vi "HW_GEN - Read Channel Default Parameters from XML File.vi"(8 "error in":errorcluster caption="错误输入（无错误）", 10 "ChanType":string="AI_QX", 11 "path to XML document":path=path "E:/00. 系统集成/!00000/11所 热气台等/SourceCodes/Builds/Files/CHdef.xml" caption="XML文档路径") -> (0 "错误输出":errorcluster, 2 "Chan dflt Para out":T3)   [LabVIEW 2016]
uses:
  Ctrls/HardWare _ Channel Configurations PopUp Type.ctl
  ToolKit/Popup/Private/Ctrls/POP_Data Type.ctl
  <vilib>/xml/Load XML File.vi
  <vilib>/xml/NI_XML.lvlib
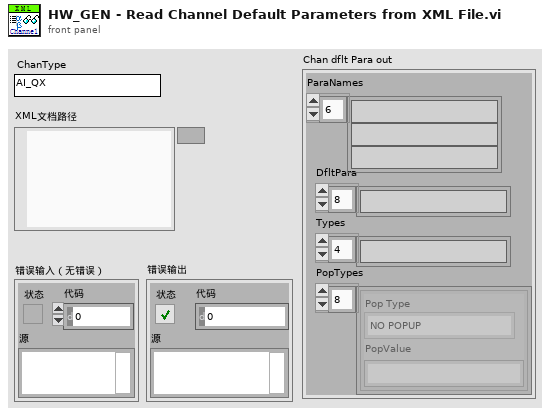
[diagram p1: front panel]
types:
  T1 = typedef "HardWare _ Channel Configurations PopUp Type.ctl" = cluster{"Pop Type":T2, "PopValue":string}
  T2 = typedef "POP_Data Type.ctl" = enum16{"NO POPUP", "Unkown", "String", "Integer", "Float", "Color", "Boolean", "Ring", "Captioned String", "Captioned Integer", "Button Color", "2 Int Cluster", "4 Int Cluster", "6-Dbl Cluster", "Path", "Combox", "Time", "ShotCut String"}
  T3 = cluster{"ParaNames":string[], "DfltPara":string[], "Types":string[], "PopTypes":T1[]}
  T4 = cluster{"Names":string[], "DfltValues":string[], "Types":string[], "PopTypes":T1[]}
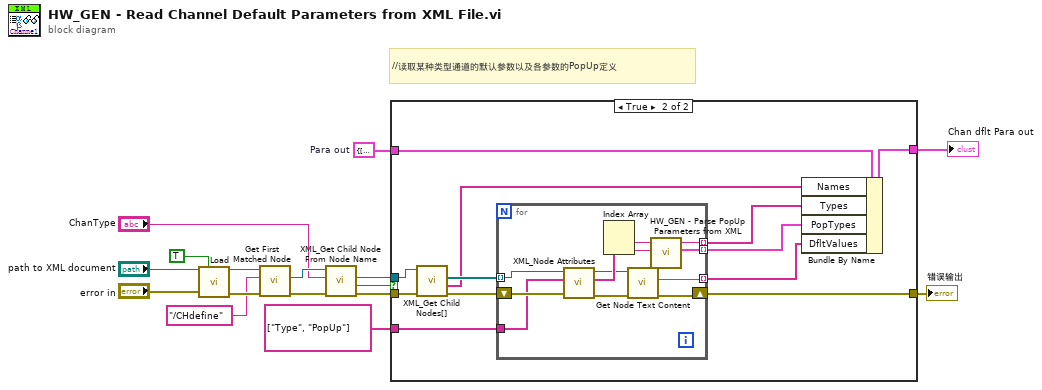
[diagram p0: block diagram]
diagram:
  w3 = T4 {"Names"=[], "DfltValues"=[], "Types"=[], "PopTypes"=[]}  # Para out
  # "//读取某种类型通道的默认参数以及各参数的PopUp定义"
  n1 = call-poly <vilib>:"Load.vi"("path to XML document"="path to XML document", "preserve whitespace (True)"=TRUE, "error in (no error)"="error in") -> ("DOM document out"=w12:refnum<k20>, "error out"=w14:errorcluster)  [unwired: 10 in, 1 out]
  n2 = call <vilib>:"Get First Matched Node.vi"("error in (no error)"=w14, "XPath expression"="/CHdefine", "node in"=w12) -> ("error out"=w10:errorcluster, "node result"=w11:refnum<k20>)  [unwired: 6 in, 1 out]
  n3 = call "XML_Get Child Node From Node Name.vi"("error in"=w10, "NodeName"="ChanType", "ref in"=w11) -> ("错误输出"=w5:errorcluster, "find?"=w7:bool, "subNode out"=w6:refnum<k20>)  [unwired: 6 in]
  n4 = case shown="True" w7 {
    tunnel: w6 -> [_ w29]
    tunnel: w5 -> [w17 w30]
    tunnel: string[] ["Type", "PopUp"] ("AttributeNames") -> [_ w26]
    tunnel: w3 -> [w18 w25]
    tunnel: [w18 w20] -> w2
    tunnel: [w17 w19] -> w1
    frame False {
    }
    frame True {
      n5 = call "XML_Get Child Nodes[].vi"("错误输入（无错误）"=w30, "ref in"=w29) -> ("错误输出"=w27:errorcluster, "NodeNames[]"=w24:string[], "ElementChildNod[]"=w28:refnum<k20>[])  [unwired: 6 in, 1 out]
      n6 = for {
        tunnel: w28 -> [w40] mode=indexing
        tunnel: w26 -> [w39]
        shift-right: [w35] -> w19
        shift-left: w27 -> [w41]
        tunnel: [w34] -> w21 mode=indexing
        tunnel: [w33] -> w23 mode=indexing
        tunnel: [w31] -> w22 mode=indexing
        n7 = call "XML_Node Attributes.vi"("error in"=w41, "AttributeNames"=w39, "node in"=w40) -> ("error out"=w36:errorcluster, "Values"=w38:string[], "node out"=w37:refnum<k20>)  [unwired: 6 in]
        n8 = Index Array(array=w38) -> (element #1=w33:string, element #2=w32:string)  [unwired: 2 in]
        n9 = call <vilib>:"Get Node Text Content.vi"("error in (no error)"=w36, "node in"=w37) -> ("error out"=w35:errorcluster, "node text"=w34:string)  [unwired: 7 in, 1 out]
        n10 = call "HW_GEN - Parse PopUp Parameters from XML.vi"("string in"=w32) -> ("PopUp"=w31:cluster{"Pop Type":T2, "string in":string})  [unwired: 10 in]
      }
      n11 = Bundle By Name(cluster=w25, "Names"=w24, "Types"=w23, "PopTypes"=w22, "DfltValues"=w21) -> (w20:T4)
    }
  }
  "Chan dflt Para out" <- w2
  "错误输出" <- w1
